vi "Preview All Messages.vi"(0 "message queue in":T3, 11 "error in":errorcluster) -> (4 "message queue out":T3, 6 "messages":T1[](array[typedef]), 15 "error out":errorcluster)   [LabVIEW 2015, in "Car Wash.lvlib" / "AMC.lvlib"]
uses:
  AMC.lvlib
  Tools/Keyed Array/KeyedArray.ctl
  Tools/Keyed Array/Tools_KeyedArray.lvlib
  Message.ctl
  Message Queue.ctl
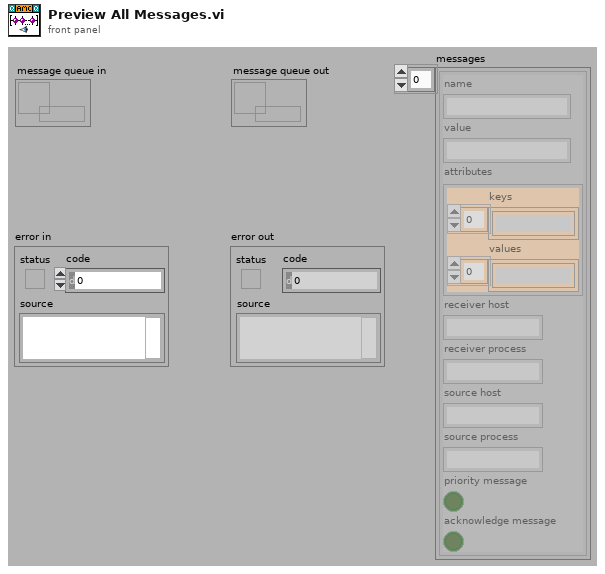
[diagram p1: front panel]
types:
  T1 = typedef "Car Wash.lvlib/AMC.lvlib/Message.ctl" = cluster{"name":string, "value":string, "attributes":T2, "receiver host":string, "receiver process":string, "source host":string, "source process":string, "priority message":bool, "acknowledge message":bool}
  T2 = typedef "Car Wash.lvlib/Tools_KeyedArray.lvlib/KeyedArray.ctl" = cluster{"keys":string[], "values":string[]}
  T3 = typedef "Car Wash.lvlib/AMC.lvlib/Message Queue.ctl" = refnum<queue>
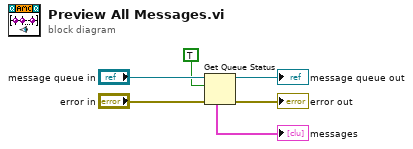
[diagram p0: block diagram]
diagram:
  n1 = Get Queue Status(queue="message queue in", return elements? (F)=TRUE, error in (no error)="error in") -> (queue out=→"message queue out":T3, error out=→"error out":errorcluster, elements=→"messages":T1[])  [unwired: 5 out]
